vi "ReadRingBlock.vi"(1 "pixel":u32=1, 2 "stop":i32, 3 "start":i32=1) -> (0 "Data Values":u16[][](graph))   [LabVIEW 2014]
uses:
  ESLSCDLL.dll
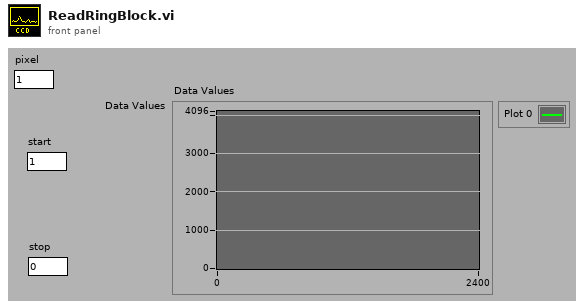
[diagram p1: front panel]
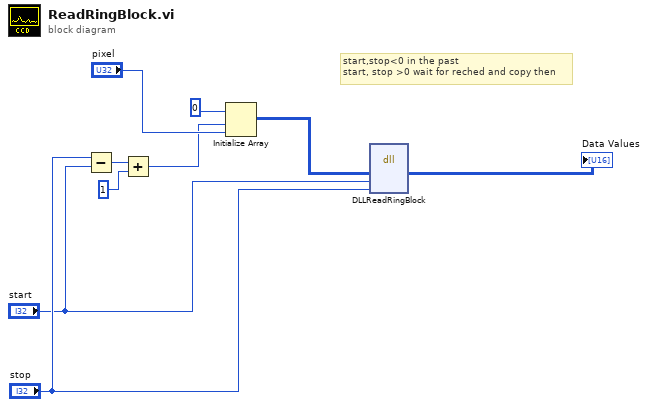
[diagram p0: block diagram]
diagram:
  # "start,stop<0 in the past\nstart, stop >0 wait for reched and copy then"
  n1 = Subtract(x="stop", y="start") -> (x-y=w5:i32)
  n2 = Add(x=w5, y=1) -> (x+y=w4:i32)
  n3 = Initialize Array(u32 0, w4, "pixel") -> (w7:u32[][])
  n4 = dll-call lib="C:/Users/Gerhard/Documents/New64/lv/1cam/board.vis/ESLSCDLL.dll" fn="DLLReadRingBlock" ("lwlscdll.dll:DLLReadLoop")("dioden"=w7, "start"="start", "stop"="stop") -> ("dioden"=→"Data Values":u16[][])  [unwired: 6 in, 2 out]
